vi "GetMaxAccTimes.vi"(8 "错误输入（无错误）":errorcluster) -> (0 "错误输出":errorcluster, 3 "返回值":u8)   [LabVIEW 2014]
uses:
  X86Dll/ZXUTConfigMgr.dll
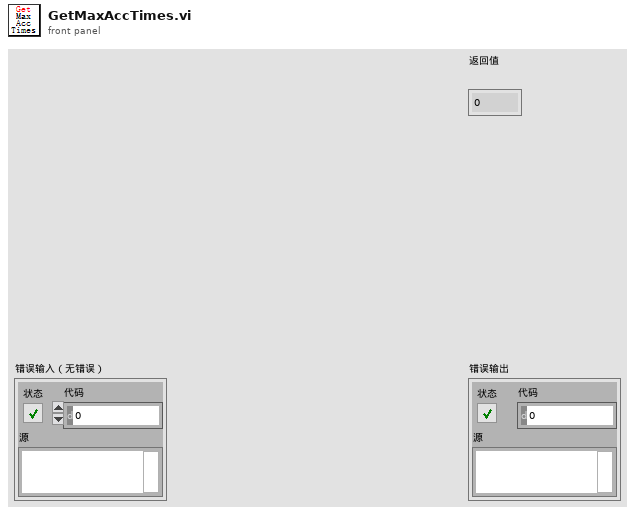
[diagram p1: front panel]
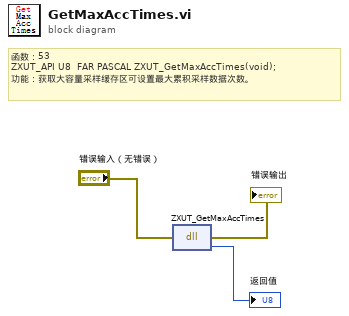
[diagram p0: block diagram]
diagram:
  # "函数：53\nZXUT_API U8\t\tFAR PASCAL ZXUT_GetMaxAccTimes(void);\n功能：获取大容量采样缓存区可设置最大累积采样数据次数。"
  n1 = dll-call lib="D:/Software/Utrasonic on-line monitoring/X86Dll/ZXUTConfigMgr.dll" fn="ZXUT_GetMaxAccTimes"(error in="错误输入（无错误）") -> (error out=→"错误输出":errorcluster, "返回值"=→"返回值":u8)  [unwired: 2 in, 1 out]
